vi "CtrlUtil.Select Tab Page by Name.vi"(2 "Name":string="Maint", 3 "Main Tab":refnum<vi>) -> ()   [LabVIEW 2024, in "EQMF.lvlib" / "Controls.lvlib"]
uses:
  Controls.lvlib
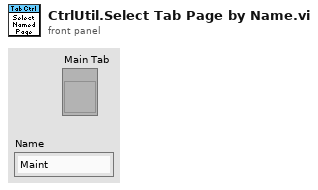
[diagram p1: front panel]
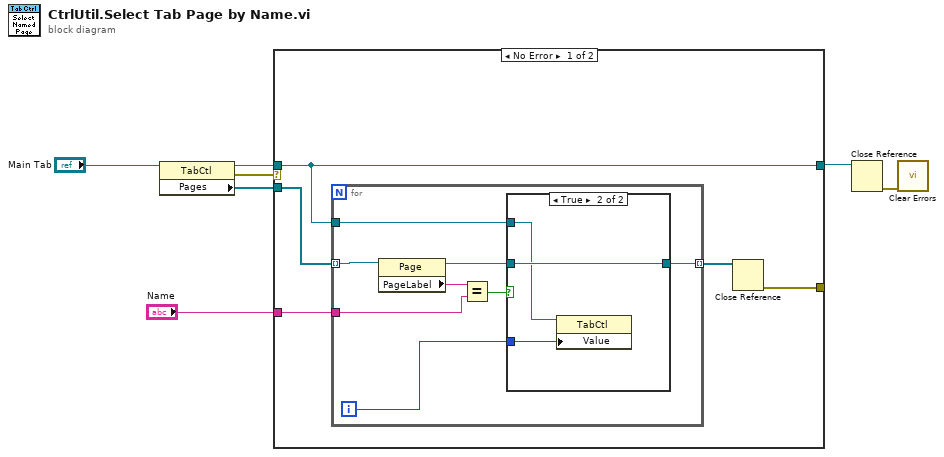
[diagram p0: block diagram]
diagram:
  n1 = property class="TabCtl"(reference="Main Tab") -> (reference out=w5:refnum<vi>, error out=w6:errorcluster, "Pages"=w7:refnum<vi>[])  [unwired: 1 in]
  n2 = case shown="No Error" w6 {
    tunnel: w7 -> [w12 _]
    tunnel: w5 -> [w9 w25]
    tunnel: [w9 w25] -> w4
    tunnel: [w10 _] -> _
    tunnel: "Name" -> [w8 _]
    frame No Error {
      n3 = for {
        tunnel: w12 -> [w20] mode=indexing
        tunnel: [w16] -> w11 mode=indexing
        tunnel: w9 -> [w15]
        tunnel: w8 -> [w13]
        i -> [w14]
        n4 = property class="Page"(reference=w20) -> (reference out=w18:refnum<vi>, "PageLabel"=w19:string)  [unwired: 1 in, 1 out]
        n5 = Equal?(x=w19, y=w13) -> (x = y?=w17:bool)
        n6 = case shown="True" w17 {
          tunnel: w18 -> [w21 w24]
          tunnel: [w21 w24] -> w16
          tunnel: w15 -> [_ w23]
          tunnel: w14 -> [_ w22]
          frame False {
          }
          frame True {
            n7 = property class="TabCtl"(reference=w23, "Value"=w22) -> ()  [unwired: 1 in, 2 out]
          }
        }
      }
      n8 = Close Reference(reference=w11) -> (error out=w10:errorcluster)  [unwired: 1 in]
    }
    frame Error {
      # "Do Nothing"
    }
  }
  n9 = Close Reference(reference=w4) -> (error out=w3:errorcluster)  [unwired: 1 in]
  n10 = call <vilib>:"Clear Errors.vi"("error in (no error)"=w3) -> ()  [unwired: 5 in, 2 out]
